vi "initTable.vi"(8 "error in":errorcluster, 10 "Column Header Strings[]":string[](array[string]), 11 "Tbl Refnum in":refnum<vi>) -> (0 "error out":errorcluster, 3 "Tbl Refnum out":refnum<vi>)   [LabVIEW 2010]
uses:
  <vilib>/Utility/miscctls.llb/LVRowAndColumnTypeDef.ctl
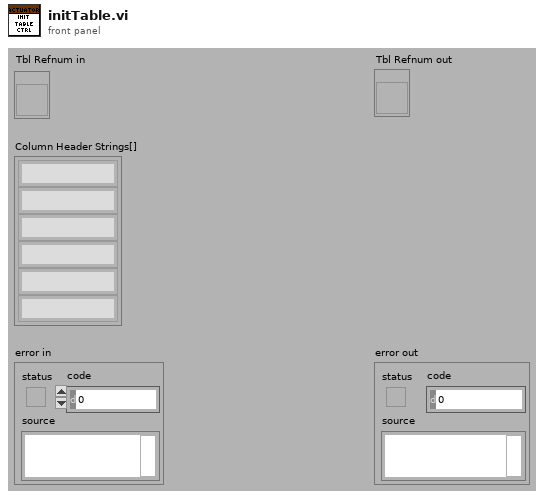
[diagram p1: front panel]
types:
  T1 = typedef "LVRowAndColumnTypeDef.ctl" = cluster{"Row":i32, "Column":i32}
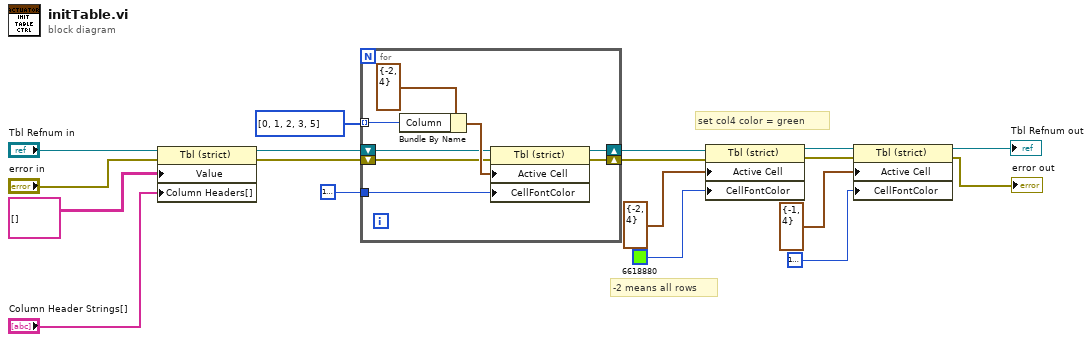
[diagram p0: block diagram]
diagram:
  # "set col4 color = green"
  # "-2 means all rows"
  n1 = property class="Tbl (strict)"(reference="Tbl Refnum in", error in="error in", "Value"=string[][] [], "Column Headers[]"="Column Header Strings[]") -> (reference out=w2:refnum<vi>, error out=w3:errorcluster)
  n2 = for {
    tunnel: i32[] [0, 1, 2, 3, 5] -> [w24] mode=indexing
    tunnel: u32 16777222 -> [w23]
    shift-right: [w22] -> w4
    shift-left: w3 -> [w20]
    shift-right: [w19] -> w1
    shift-left: w2 -> [w21]
    n3 = Bundle By Name(cluster=T1 {"Row"=-2, "Column"=4} ("Active Cell:Active Cell"), "Column"=w24) -> (w25:T1)
    n4 = property on="Property Node" class="Tbl (strict)"(reference=w21, error in=w20, "Active Cell"=w25, "CellFontColor"=w23) -> (reference out=w19:refnum<vi>, error out=w22:errorcluster)
  }
  n5 = property on="Property Node" class="Tbl (strict)"(reference=w1, error in=w4, "Active Cell"=T1 {"Row"=-2, "Column"=4} ("Active Cell:Active Cell"), "CellFontColor"=u32 6618880) -> (reference out=w12:refnum<vi>, error out=w11:errorcluster)
  n6 = property on="Property Node" class="Tbl (strict)"(reference=w12, error in=w11, "Active Cell"=T1 {"Row"=-1, "Column"=4} ("Active Cell:Active Cell"), "CellFontColor"=u32 16777222) -> (reference out=→"Tbl Refnum out":refnum<vi>, error out=→"error out":errorcluster)
